vi "Packet Encode.vi"(8 "error in (no error)":errorcluster, 11 "Score in":refnum<class "Score.lvclass">) -> (0 "error out":errorcluster, 2 "Data":u8[](array[numeric]), 3 "Score out":refnum<class "Score.lvclass">)   [LabVIEW 2019, in "Score.lvclass"]
uses:
  Score.lvclass
  TCP Packet/Packet.lvclass
  PlayerUpdate/PlayerUpdate.lvclass
  C:/projects/labview_multiplayer_snake/Main Codeline/Software/Code/Shared/PlayerUpdate/PlayerUpdate.lvclass
  C:/projects/labview_multiplayer_snake/Main Codeline/Software/Code/Shared/TCP/JSONPayload/JSONPayload.lvclass
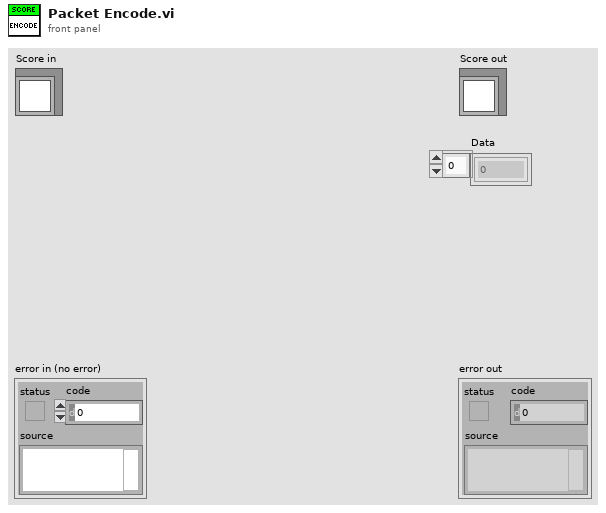
[diagram p1: front panel]
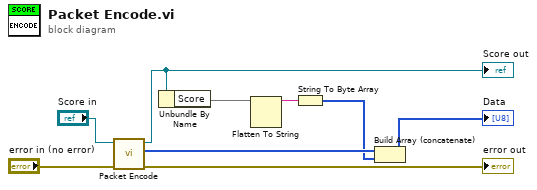
[diagram p0: block diagram]
diagram:
  n1 = call-parent "Packet Encode.vi"("error in (no error)"="error in (no error)", "Packet in"="Score in") -> ("error out"=→"error out":errorcluster, "Data"=w3:u8[], "Packet out"=w6:refnum<class "Packet.lvclass">)  [unwired: 7 in]
  "Score out" <- w6
  n2 = Unbundle By Name(w6) -> ("Score"=w5)
  n3 = Flatten To String(anything=w5) -> (data string=w4:string)  [unwired: 3 in, 2 out]
  n4 = String To Byte Array(string=w4) -> (unsigned byte array=w2:u8[])
  n5 = Build Array (concatenate)(w3, w2) -> (→"Data":u8[])
